vi "SG_Example.vi"() -> ()   [LabVIEW 2016]
uses:
  Source/SG/Typedefs/Waveform Timing Configuration.ctl
  <instrlib>/niRFSG/niRFSG.llb/niRFSG Exported Signal Destinations.ctl
  Source/SG/Typedefs/PAEN Configuration.ctl
  <instrlib>/niRFSG/niRFSG.llb/niRFSG Ref Clock Sources.ctl
  Source/Common/Local Oscillator Sharing Mode.ctl
  Source/SG/Typedefs/Instrument Configuration.ctl
  Source/SG/SG.lvlib
  Source/Common/Common.lvlib
panel:
  in  "Configurations":enum32{"General", "Generation Configuration"}(tab)
  in  "resource name":refnum<k15>
  in  "Waveform File Path":path=path "C:/Users/Public/Documents/National Instruments/RFIC Test Software/Waveforms/NR_FR1_UL_1x100MHz_30kHz-SCS_256QAM_OS4_VST2_1ms.tdms"
  in  "Carrier Frequency (Hz)":dbl=3500000000.0 format="%#_6p"
  in  "DUT Average Input Power (dBm)":dbl=-10.0
  in  "External Attenuation (dB)":dbl
  in  "Reference Clock Source":T1="PXI_CLK"
  in  "LO Sharing Mode":T2
  in  "SelectedPorts":string
  in  "Generation Mode":enum32{"Continuous", "Bursted"}(tab)
  in  "Waveform Start Trigger Export":T3="PXI_Trig0"
  in  "Waveform Timing Configuration":T4={"Duty Cycle (%)"=50.0, "Pre-Burst Time (s)"=1e-06, "Post-Burst Time (s)"=1e-06, "Burst Start Trigger Export"="PXI_Trig0"} {"Post-Burst Time (s)" format="%#_6p"; "Pre-Burst Time (s)" format="%#_6p"; "Duty Cycle (%)" min=1.0 max=100.0 step=1.0 format="%#_2d%%"}
  in  "PAEN Configuration":T5={"PAEN Mode"=enum."Dynamic", "PA Enable Trigger Export Terminal"="PFI0", "PA Enable Trigger Mode"=23001, "Command Enable Time (s)"=0.0, "Command Disable Time (s)"=0.0} {"PA Enable Trigger Mode" items=["Pulse"=23000, "Toggle"=23001]; "Command Disable Time (s)" format="%#_6p"; "Command Enable Time (s)" format="%#_6p"}
  in  "stop":bool
  out "Status":string
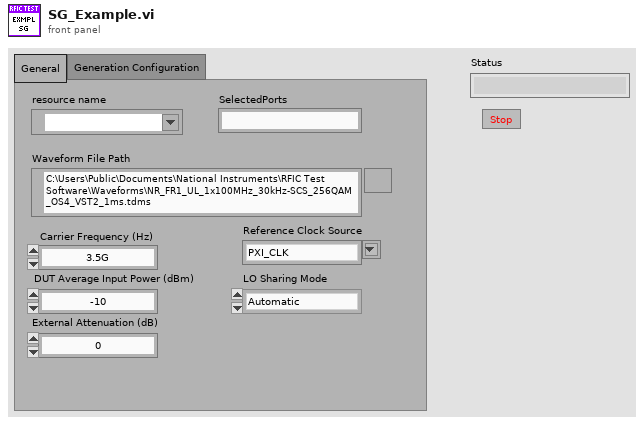
[diagram p1: front panel]
types:
  T1 = typedef "niRFSG Ref Clock Sources.ctl" = string
  T2 = typedef "Common.lvlib/Local Oscillator Sharing Mode.ctl" = enum16{"Automatic", "None"}
  T3 = typedef "niRFSG Exported Signal Destinations.ctl" = string
  T4 = typedef "SG.lvlib/Waveform Timing Configuration.ctl" = cluster{"Duty Cycle (%)":dbl, "Pre-Burst Time (s)":dbl, "Post-Burst Time (s)":dbl, "Burst Start Trigger Export":T3}
  T5 = typedef "SG.lvlib/PAEN Configuration.ctl" = cluster{"PAEN Mode":enum16{"Disabled", "Static", "Dynamic"}, "PA Enable Trigger Export Terminal":T3, "PA Enable Trigger Mode":i32, "Command Enable Time (s)":dbl, "Command Disable Time (s)":dbl}
  T6 = typedef "SG.lvlib/Instrument Configuration.ctl" = cluster{"SelectedPorts":string, "Reference Clock Source":T1, "Carrier Frequency (Hz)":dbl, "DUT Average Input Power (dBm)":dbl, "External Attenuation (dB)":dbl, "LO Sharing Mode":T2}
  T7 = typedef "Common.lvlib/Waveform.ctl" = cluster{"Name":string, "Data":refnum<data-value>, "Signal Bandwidth (Hz)":dbl, "PAPR (dB)":dbl, "Burst Length (s)":dbl, "Sample Rate":dbl, "Burst Start Locations":i32[], "Burst Stop Locations":i32[], "Idle Duration Present?":bool, "Runtime Scaling":dbl, "Script":string}
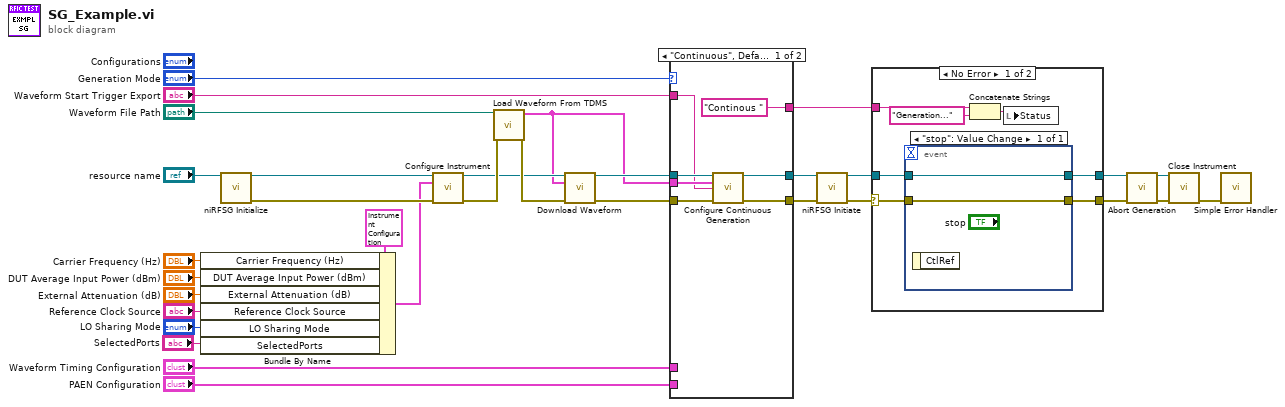
[diagram p0: block diagram]
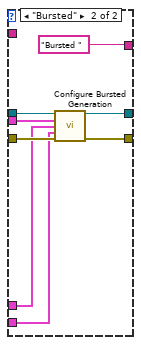
[diagram p2: hidden frame]
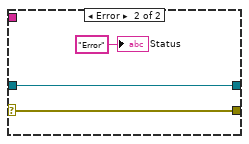
[diagram p3: hidden frame]
diagram:
  n1 = Bundle By Name(cluster=T6 {"SelectedPorts"="", "Reference Clock Source"="OnboardClock", "Carrier Frequency (Hz)"=1000000000.0, "DUT Average Input Power (dBm)"=-20.0, "External Attenuation (dB)"=0.0, "LO Sharing Mode"=enum."Automatic"} ("SG Configuration"), "Carrier Frequency (Hz)"="Carrier Frequency (Hz)", "DUT Average Input Power (dBm)"="DUT Average Input Power (dBm)", "External Attenuation (dB)"="External Attenuation (dB)", "Reference Clock Source"="Reference Clock Source", "LO Sharing Mode"="LO Sharing Mode", "SelectedPorts"="SelectedPorts") -> (w7:T6)
  n2 = call <instrlib>:"niRFSG Initialize.vi"("resource name"="resource name") -> ("instrument handle"=w26:refnum<k15>, "error out"=w32:errorcluster)  [unwired: 13 in]
  n3 = call "Configure Instrument.vi"("RFSG Session In"=w26, "SG Configuration"=w7, "error in (no error)"=w32) -> ("RFSG Session Out"=w23:refnum<k15>, "error out"=w28:errorcluster)  [unwired: 11 in]
  n4 = call "Load Waveform From TDMS.vi"("TDMS File Path"="Waveform File Path", "error in (no error)"=w28) -> ("Waveform"=w21:T7, "error out"=w27:errorcluster)  [unwired: 12 in]
  n5 = call "Download Waveform.vi"("RFSG handle"=w23, "Waveform In"=w21, "error in (no error)"=w27) -> ("RFSG handle out"=w22:refnum<k15>, "error out"=w29:errorcluster)  [unwired: 11 in]
  n6 = case shown="\"Continuous\", Default" "Generation Mode" {
    tunnel: [w38 w47] -> w31
    tunnel: w29 -> [w39 w46]
    tunnel: [w36 w45] -> w25
    tunnel: w22 -> [w37 w44]
    tunnel: w21 -> [w35 w43]
    tunnel: "Waveform Timing Configuration" -> [_ w42]
    tunnel: "PAEN Configuration" -> [_ w41]
    tunnel: "Waveform Start Trigger Export" -> [w34 _]
    tunnel: ["Continous " "Bursted "] -> w2
    frame "Continuous", Default {
      n7 = call "Configure Continuous Generation.vi"("RFSG handle"=w37, "Waveform in"=w35, "Waveform Start Trigger Export"=w34, "error in"=w39) -> ("RFSG handle out"=w36:refnum<k15>, "error out"=w38:errorcluster)  [unwired: 9 in, 1 out]
    }
    frame "Bursted" {
      n8 = call "Configure Bursted Generation.vi"("RFSG handle"=w44, "Waveform"=w43, "Waveform Timing Configuration"=w42, "PAEN Configuration"=w41, "error in"=w46) -> ("RFSG handle out"=w45:refnum<k15>, "error out"=w47:errorcluster)  [unwired: 7 in, 2 out]
    }
  }
  n9 = call <instrlib>:"niRFSG Initiate.vi"("instrument handle"=w25, "error in"=w31) -> ("instrument handle out"=w18:refnum<k15>, "error out"=w13:errorcluster)  [unwired: 12 in]
  n10 = case shown="No Error" w13 {
    selector: w13 -> [w50 w59]
    tunnel: w18 -> [w54 w58]
    tunnel: [w53 w58] -> w17
    tunnel: [w52 w59] -> w16
    tunnel: w2 -> [w48 _]
    frame No Error {
      n11 = event shown="[0] \"stop\": Value Change" {
        selector: _ -> [_]
        dyn-events: _ -> [_]
        timeout: _ -> [_]
        tunnel: w50 -> [w55]
        tunnel: w54 -> [w56]
        tunnel: [w56] -> w53
        tunnel: [w55] -> w52
        event "stop": Value Change {
          n12 = event-data() -> ()  [unwired: 1 in, 1 out]
        }
      }
      n13 = Concatenate Strings(w48, "Generation..." ("Status")) -> (w49:string)
      n14 = local write "Status"(w49) -> ()
    }
    frame Error {
      "Status" <- "Error" ("Status")
    }
  }
  n15 = call "Abort Generation.vi"("RFSG handle"=w17, "error in (no error)"=w16) -> ("RFSG handle out"=w24:refnum<k15>, "error out"=w30:errorcluster)  [unwired: 12 in]
  n16 = call "Close Instrument.vi"("RFSG Handle"=w24, "error in (no error)"=w30) -> ("error out"=w15:errorcluster)  [unwired: 13 in]
  n17 = call <vilib>:"Simple Error Handler.vi"("error in (no error)"=w15) -> ()  [unwired: 4 in, 5 out]
